vi "listboxReplaceElement.vi"(7 "inElement":string="track_positions", 8 "error in (no error)":errorcluster, 9 "replaceElementWith":string, 10 "elementName":string, 11 "TabCtl Refnum":refnum<vi>) -> (0 "error out":errorcluster, 3 "TabCtl Refnum out":refnum<vi>)   [LabVIEW 2009, in "Views.lvlib" / "Camera.lvlib" / "andorSettingsViewer.lvclass"]
uses:
  andorSettingsViewer.lvclass
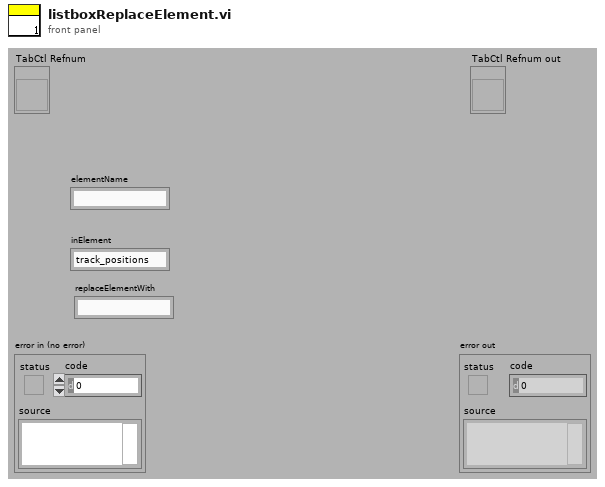
[diagram p1: front panel]
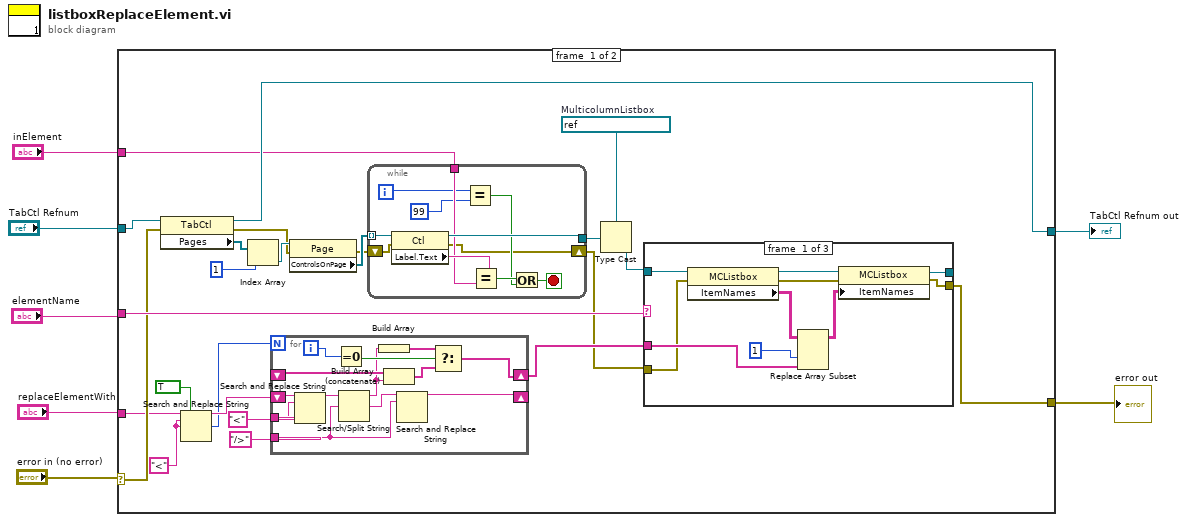
[diagram p0: block diagram]
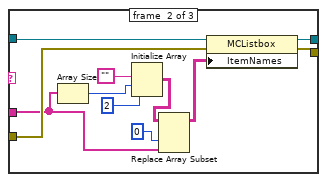
[diagram p2: hidden frame]
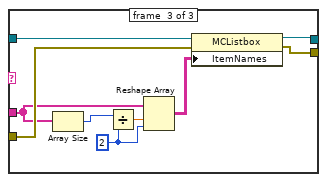
[diagram p3: hidden frame]
diagram:
  n1 = case shown="No Error" "error in (no error)" {
    selector: "error in (no error)" -> [w11 w86]
    tunnel: [w14 w86] -> w6
    tunnel: "TabCtl Refnum" -> [w31 _]
    tunnel: [w30 _] -> w4
    tunnel: "elementName" -> [w29 _]
    tunnel: "inElement" -> [w9 _]
    tunnel: "replaceElementWith" -> [w8 _]
    frame #0 {
      w15 = refnum<vi> refnum  # MulticolumnListbox
      w28 = "<"
      n2 = property class="TabCtl"(reference=w31, error in=w11) -> (reference out=w30:refnum<vi>, error out=w12:errorcluster, "Pages"=w21:refnum<vi>[])
      n3 = Search and Replace String(replace all?=TRUE, input string=w8, search string=w28, replace string=w28) -> (result string=w24:string, number of replacements=w22:i32)  [unwired: 4 in, 2 out]
      n4 = Index Array(array=w21, index=1) -> (element=w19:refnum<vi>)
      n5 = for {
        N: w22 -> [_]
        tunnel: "<" -> [w83]
        tunnel: "/>" -> [w80]
        shift-right: [w79] -> _
        shift-left: w24 -> [w84]
        shift-right: [w75] -> w23
        shift-left: _ -> [w82]
        i -> [w78]
        n6 = Search and Replace String(input string=w84, search string=w83) -> (result string=w85:string)  [unwired: 6 in, 3 out]
        n7 = Equal To 0?(x=w78) -> (x = 0?=w77:bool)
        n8 = Search/Split String(string=w85, search string/char (-)=w80) -> (substring before match=w73:string, match + rest of string=w81:string)  [unwired: 1 in, 1 out]
        n9 = Build Array(w73) -> (w74:string[])
        n10 = Build Array (concatenate)(w82, w73) -> (w76:string[])
        n11 = Search and Replace String(input string=w81, search string=w80) -> (result string=w79:string)  [unwired: 6 in, 3 out]
        n12 = Select(t=w74, s=w77, f=w76) -> (s? t:f=w75:string[])
      }
      n13 = property class="Page"(reference=w19, error in=w12) -> (error out=w13:errorcluster, "ControlsOnPage"=w18:refnum<vi>[])  [unwired: 1 out]
      n14 = while {
        tunnel: w18 -> [w72] mode=indexing
        tunnel: w9 -> [w68]
        tunnel: [w69] -> w16
        shift-right: [w63] -> w10
        shift-left: w13 -> [w62]
        i -> [w67]
        stop <- w65 stop-if-true
        n15 = property class="Ctl"(reference=w72, error in=w62) -> (reference out=w69:refnum<vi>, error out=w63:errorcluster, "Label.Text"=w70:string)
        n16 = Equal?(x=w67, y=99) -> (x = y?=w64:bool)
        n17 = Equal?(x=w70, y=w68) -> (x = y?=w71:bool)
        n18 = Or(x=w71, y=w64) -> (x .or. y?=w65:bool)
      }
      n19 = Type Cast(type=w15, x=w16) -> (*(type *) &x=w17:refnum<vi>)
      n20 = case shown="\"top\"" w29 {
        tunnel: w23 -> [w38 w45 w57]
        tunnel: w17 -> [w37 w47 w59]
        tunnel: w10 -> [w34 w46 w58]
        tunnel: [w39 w52 w61] -> _
        tunnel: [w40 w51 w60] -> w14
        frame #0 {
          n21 = property class="MCListbox"(reference=w37, error in=w34) -> (reference out=w36:refnum<vi>, error out=w35:errorcluster, "ItemNames"=w33:string[][])
          n22 = Replace Array Subset(array=w33, new element=w38, index (col)=1) -> (w41:string[][])  [unwired: 1 in]
          n23 = property class="MCListbox"(reference=w36, error in=w35, "ItemNames"=w41) -> (reference out=w39:refnum<vi>, error out=w40:errorcluster)
        }
        frame #1 {
          n24 = Array Size(array=w45) -> (size(s)=w43:i32)
          n25 = Initialize Array("", w43, 2) -> (w49:string[][])
          n26 = Replace Array Subset(array=w49, new element=w45, index (col)=0) -> (w48:string[][])  [unwired: 1 in]
          n27 = property class="MCListbox"(reference=w47, error in=w46, "ItemNames"=w48) -> (reference out=w52:refnum<vi>, error out=w51:errorcluster)
        }
        frame #2 {
          w56 = 2
          n28 = Array Size(array=w57) -> (size(s)=w55:i32)
          n29 = Divide(x=w55, y=w56) -> (x/y=w54:dbl)
          n30 = Reshape Array(w57, w54, w56) -> (w53:string[][])
          n31 = property class="MCListbox"(reference=w59, error in=w58, "ItemNames"=w53) -> (reference out=w61:refnum<vi>, error out=w60:errorcluster)
        }
      }
    }
    frame #1 {
    }
  }
  "error out" <- w6
  "TabCtl Refnum out" <- w4
